vi "emergency.vi"   [LabVIEW 2013]
uses:
  FT_HMI.llb/GLOBAL_GEN.vi
  ADS.llb/Global DIOs.vi
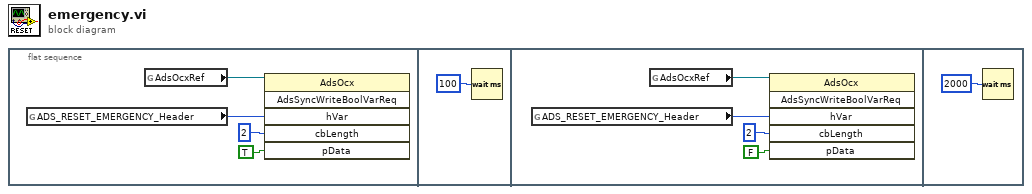
[diagram p0: block diagram]
diagram:
  n1 = flat-sequence {
    frame #0 {
      n2 = global read "Global DIOs.vi" "ADS_RESET_EMERGENCY_Header"() -> (w1:i32)
      n3 = global read "GLOBAL_GEN.vi" "AdsOcxRef"() -> (w2:refnum<k7>)
      n4 = invoke class="AdsOcx" method="AdsSyncWriteBoolVarReq"(reference=w2, "hVar"=w1, "cbLength"=2 ("phConnect"), "pData"=TRUE) -> ()  [unwired: 2 in, 6 out]
    }
    frame #1 {
      n5 = Wait (ms)(milliseconds to wait=u32 100) -> ()  [unwired: 1 out]
    }
    frame #2 {
      n6 = global read "Global DIOs.vi" "ADS_RESET_EMERGENCY_Header"() -> (w6:i32)
      n7 = global read "GLOBAL_GEN.vi" "AdsOcxRef"() -> (w7:refnum<k7>)
      n8 = invoke class="AdsOcx" method="AdsSyncWriteBoolVarReq"(reference=w7, "hVar"=w6, "cbLength"=2 ("phConnect"), "pData"=FALSE) -> ()  [unwired: 2 in, 6 out]
    }
    frame #3 {
      n9 = Wait (ms)(milliseconds to wait=u32 2000) -> ()  [unwired: 1 out]
    }
  }
